vi "Shutdown.vi"(8 "error in (no error)":errorcluster, 11 "Controller in":refnum<class "Controller.lvclass">) -> (0 "error out":errorcluster, 3 "Controller out":refnum<class "Controller.lvclass">)   [LabVIEW 2013, in "SET Project Editor.lvlib" / "Controller.lvclass"]
uses:
  Controller.lvclass
  Controller.lvclass/Controller.ctl
  <vilib>/ActorFramework/Actor/Actor.lvclass/Actor.ctl
  <vilib>/ActorFramework/Message Enqueuer/Message Enqueuer.lvclass/Message Enqueuer.ctl
  <vilib>/ActorFramework/Message Enqueuer/Init from Existing Queue.vi
  <vilib>/ActorFramework/Message Enqueuer/Enqueue.vi
  <vilib>/ActorFramework/Message Priority Queue/Priority Enqueue.vi
  <vilib>/ActorFramework/Message Enqueuer/Message Enqueuer.lvclass
  <vilib>/ActorFramework/Stop Msg/Stop Msg.lvclass
  <vilib>/ActorFramework/Actor/Actor.lvclass
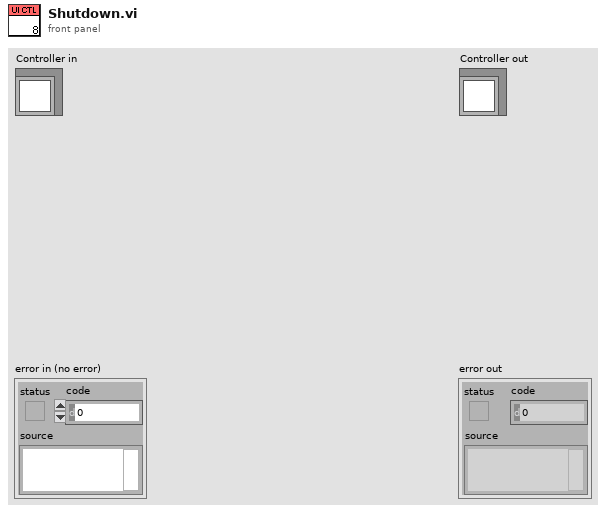
[diagram p1: front panel]
types:
  T1 = enum16{"Left Button", "Center Button", "Right Button", "Window Close"}
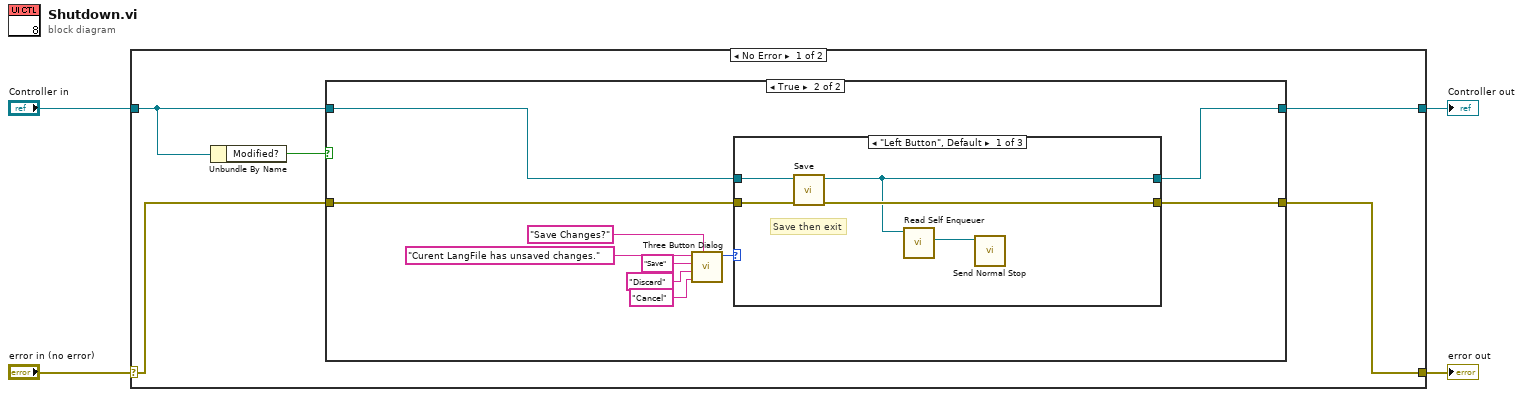
[diagram p0: block diagram]
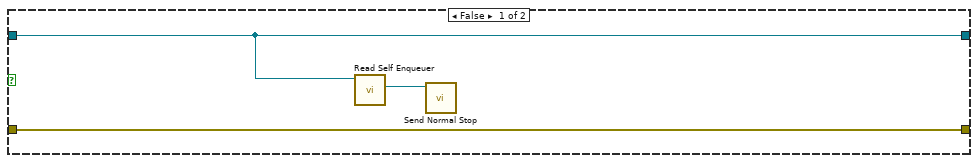
[diagram p2: hidden frame]
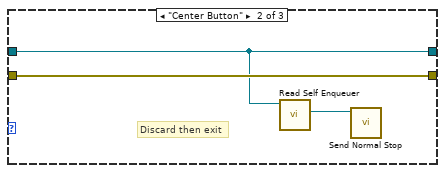
[diagram p3: hidden frame]
diagram:
  n1 = case shown="No Error" "error in (no error)" {
    selector: "error in (no error)" -> [w6 w34]
    tunnel: [w5 w34] -> w3
    tunnel: [w7 w33] -> w1
    tunnel: "Controller in" -> [w8 w33]
    frame No Error {
      n2 = Unbundle By Name(w8) -> ("Modified?"=w9:bool)
      n3 = case shown="True" w9 {
        tunnel: w8 -> [w10 w16]
        tunnel: [w10 w15] -> w7
        tunnel: w6 -> [w12 w13]
        tunnel: [w12 w14] -> w5
        frame False {
          n4 = call <vilib>:"Read Self Enqueuer.vi"("Actor"=w10) -> ("Self Enqueuer"=w11:refnum<class "Message Enqueuer.lvclass">)  [unwired: 10 in]
          n5 = call <vilib>:"Send Normal Stop.vi"("Message Enqueuer"=w11) -> ()  [unwired: 10 in, 1 out]
        }
        frame True {
          n6 = call <vilib>:"Three Button Dialog.vi"("Window Title (\"\")"="Save Changes?" ("Window Title (\"\")"), "Right Button Text (\"Cancel\")"="Cancel" ("Right Button Text (\"Cancel\")"), "Center Button Text (\"No\")"="Discard" ("Center Button Text (\"No\")"), "Left Button Text (\"Yes\")"="Save" ("Left Button Text (\"Yes\")"), "message"="Curent LangFile has unsaved changes.") -> ("Which Button?"=w22:T1)  [unwired: 6 in]
          n7 = case shown="\"Left Button\", Default" w22 {
            tunnel: w16 -> [w27 w28 w32]
            tunnel: [w24 w28 w32] -> w15
            tunnel: w13 -> [w26 w30 w31]
            tunnel: [w25 w30 w31] -> w14
            frame "Left Button", Default {
              # "Save then exit"
              n8 = call-dynamic "Save.vi"("error in (no error)"=w26, "Controller in"=w27) -> ("error out"=w25:errorcluster, "Controller out"=w24:refnum<class "Controller.lvclass">)  [unwired: 8 in]
              n9 = call <vilib>:"Read Self Enqueuer.vi"("Actor"=w24) -> ("Self Enqueuer"=w23:refnum<class "Message Enqueuer.lvclass">)  [unwired: 10 in]
              n10 = call <vilib>:"Send Normal Stop.vi"("Message Enqueuer"=w23) -> ()  [unwired: 10 in, 1 out]
            }
            frame "Center Button" {
              # "Discard then exit"
              n11 = call <vilib>:"Read Self Enqueuer.vi"("Actor"=w28) -> ("Self Enqueuer"=w29:refnum<class "Message Enqueuer.lvclass">)  [unwired: 10 in]
              n12 = call <vilib>:"Send Normal Stop.vi"("Message Enqueuer"=w29) -> ()  [unwired: 10 in, 1 out]
            }
            frame "Right Button" {
              # "Don't Exit"
            }
          }
        }
      }
    }
    frame Error {
    }
  }
  "error out" <- w3
  "Controller out" <- w1
